vi "Set Components.vi"(8 "error in (no error)":errorcluster, 10 "Components":refnum<class "Component.lvclass">[](array[class]), 11 "Item Ref in":T1 format="%.0x") -> (0 "error out":errorcluster, 3 "Item Ref out":T1 format="%.0x")   [LabVIEW 2017, in "DSF System Explorer.lvlib"]
uses:
  DSF System Explorer.lvlib
  <vilib>/NI Veristand/Custom Device API/Custom Device Item Ref.ctl
  DSF Core.lvlibp/Classes/Component/Component.lvclass
  Components Ref.ctl
  Components.ctl
  <vilib>/NI Veristand/Custom Device API/Get Item Property (U32).vi
  <vilib>/NI Veristand/Custom Device API/Custom Device API.lvlib
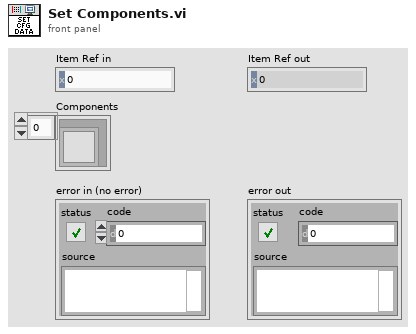
[diagram p1: front panel]
types:
  T1 = typedef "Custom Device API.lvlib/Custom Device Item Ref.ctl" = u64
  T2 = typedef "DSF System Explorer.lvlib/Components Ref.ctl" = refnum<data-value>
  T3 = typedef "DSF System Explorer.lvlib/Components.ctl" = cluster{"Components":refnum<class "Component.lvclass">[]}
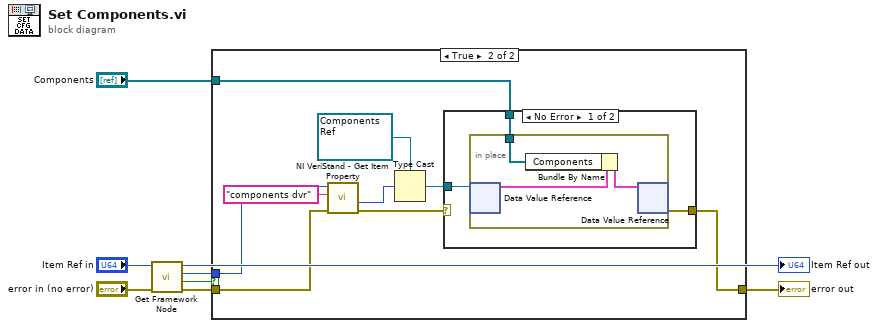
[diagram p0: block diagram]
diagram:
  n1 = call "Get Framework Node.vi"("error in (no error)"="error in (no error)", "Item Ref in"="Item Ref in") -> ("error out"=w6:errorcluster, "found?"=w3:bool, "Framework Ref"=w5:T1, "Item Ref out"=→"Item Ref out":T1)  [unwired: 6 in]
  n2 = case shown="True" w3 {
    tunnel: w6 -> [w9 w14]
    tunnel: w5 -> [_ w13]
    tunnel: [w9 w12] -> w4
    tunnel: "Components" -> [_ w10]
    frame False {
    }
    frame True {
      n3 = call-poly <vilib>:"NI VeriStand - Get Item Property.vi"("error in (no error)"=w14, "Property Name"="components dvr", "Item Ref in"=w13) -> ("error out"=w15:errorcluster, "Value"=w17:u32)  [unwired: 5 in, 2 out]
      n4 = Type Cast(type=T2 refnum ("data value reference"), x=w17) -> (*(type *) &x=w16:T2)
      n5 = case shown="No Error" w15 {
        selector: w15 -> [_ w25]
        tunnel: w16 -> [w21 _]
        tunnel: [w20 w25] -> w12
        tunnel: w10 -> [w19 _]
        frame No Error {
          n6 = in-place {
            in-place-border: w19 -> [w22]
            n7 = in-place-dvr #1(w21) -> (w24:T3)  [unwired: 1 out]
            n8 = Bundle By Name(cluster=w24, "Components"=w22) -> (w23:T3)
            n9 = in-place-dvr #1(w23) -> (w20:errorcluster)  [unwired: 1 out]
          }
        }
        frame Error {
        }
      }
    }
  }
  "error out" <- w4
